vi "Write Arr of Channel Ref.vi"(8 "error in (no error)":errorcluster, 10 "Arr of Channel Ref":refnum<vi>, 11 "Generic Data Logger Card in":refnum<class "Generic Data Logger Card.lvclass">) -> (0 "error out":errorcluster, 3 "Generic Data Logger Card out":refnum<class "Generic Data Logger Card.lvclass">)   [LabVIEW 2013, in "Generic Data Logger.lvlib" / "Generic Data Logger Card.lvclass"]
uses:
  Generic Data Logger Card.lvclass
  Generic Data Logger Card.lvclass/Generic Data Logger Card.ctl
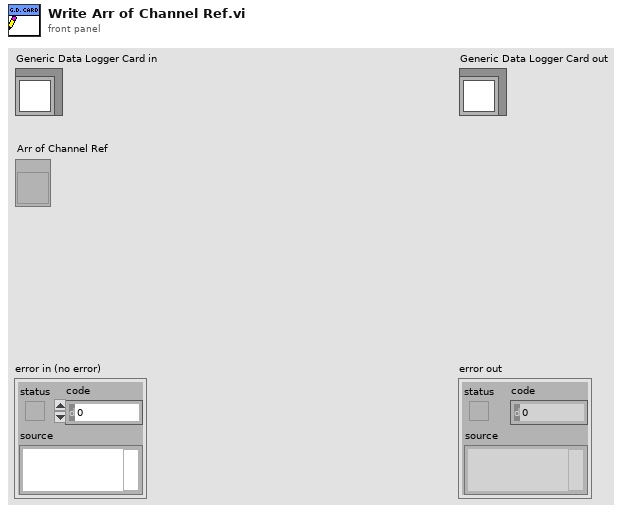
[diagram p1: front panel]
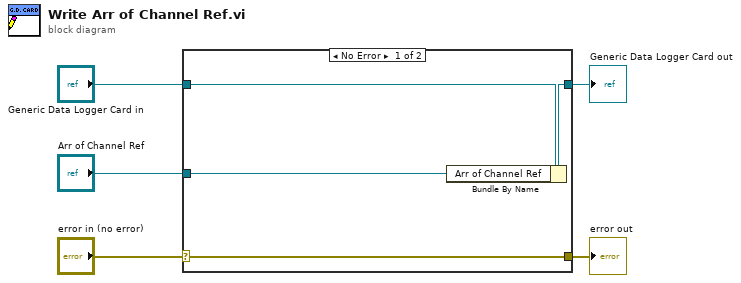
[diagram p0: block diagram]
diagram:
  n1 = case shown="No Error" "error in (no error)" {
    selector: "error in (no error)" -> [w9 w10]
    tunnel: [w9 w10] -> w4
    tunnel: [w7 w11] -> w2
    tunnel: "Generic Data Logger Card in" -> [w8 w11]
    tunnel: "Arr of Channel Ref" -> [w6 _]
    frame No Error {
      n2 = Bundle By Name(cluster=w8, "Arr of Channel Ref"=w6) -> (w7:refnum<class "Generic Data Logger Card.lvclass">)
    }
    frame Error {
    }
  }
  "error out" <- w4
  "Generic Data Logger Card out" <- w2
